vi "Sprache bei den Elementen aendern.vi"(7 "Index":i32, 8 "Fehler (Eingang, kein Fehler)":errorcluster, 9 "Sprachauswahl":u16, 10 "Index verwenden":bool, 11 "VI Referenzen":refnum<vi>[](array[refnum])) -> (0 "Fehler (Ausgang)":errorcluster, 6 "KlassenID":u32[][](array[numeric]))   [LabVIEW 2020, in "Sprachverwaltung.lvlib"]
uses:
  Sprachverwaltung.lvlib
  FGV Aktion Tabelle zerlegen.ctl
panel:
  # "3 Generic \n4 Decoration \n5 Text \n6 Control \n7 ColorBox \n8 Boolean \n9 RefNum \n10 Variant \n11 Path \n12 ListBox \n13 Table \n14 Array \n15 Picture \n16 ActiveXContainer \n17 Numeric \n18 Digital \n19 NamedNumeric \n20 ColorRamp \n21 Slide \n22 GraphOrChart \n23 WaveformChart \n24 WaveformGraph \n25 IntensityChart \n26 IntensityGraph \n27 String \n28 IOName \n29 ComboBox \n30 Cluster \n31 Panel \n32 Knob \n33 NumWithScale \n34 Ring \n35 Enum \n36 GObject \n37 Plot \n38 Cursor \n39 NumericText \n40 Scale \n41 ColorScale \n42 GraphScale \n43 ColorGraphScale \n44 TypedRefNum \n45 OldKnobScale \n46 MCListbox \n47 MeasureData \n48 BVTag \n49 DAQName \n50 VISAName \n51 IVIName \n52 SlideScale \n54 Page \n55 TabControl \n56 ConPane"
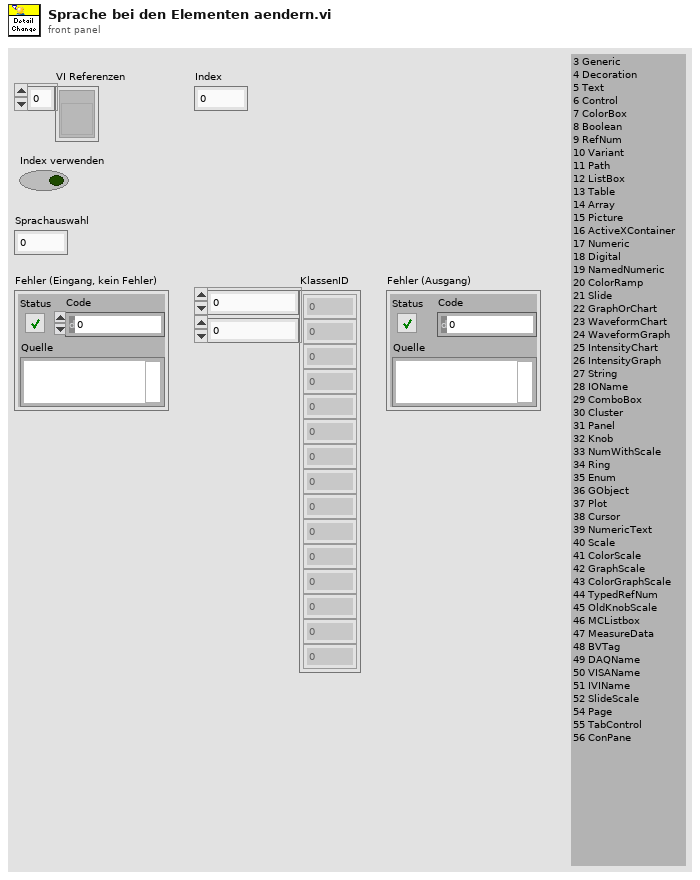
[diagram p1: front panel]
types:
  T1 = typedef "Sprachverwaltung.lvlib/FGV Aktion Tabelle zerlegen.ctl" = enum16{"laden", "vereinzeln", "speichern"}
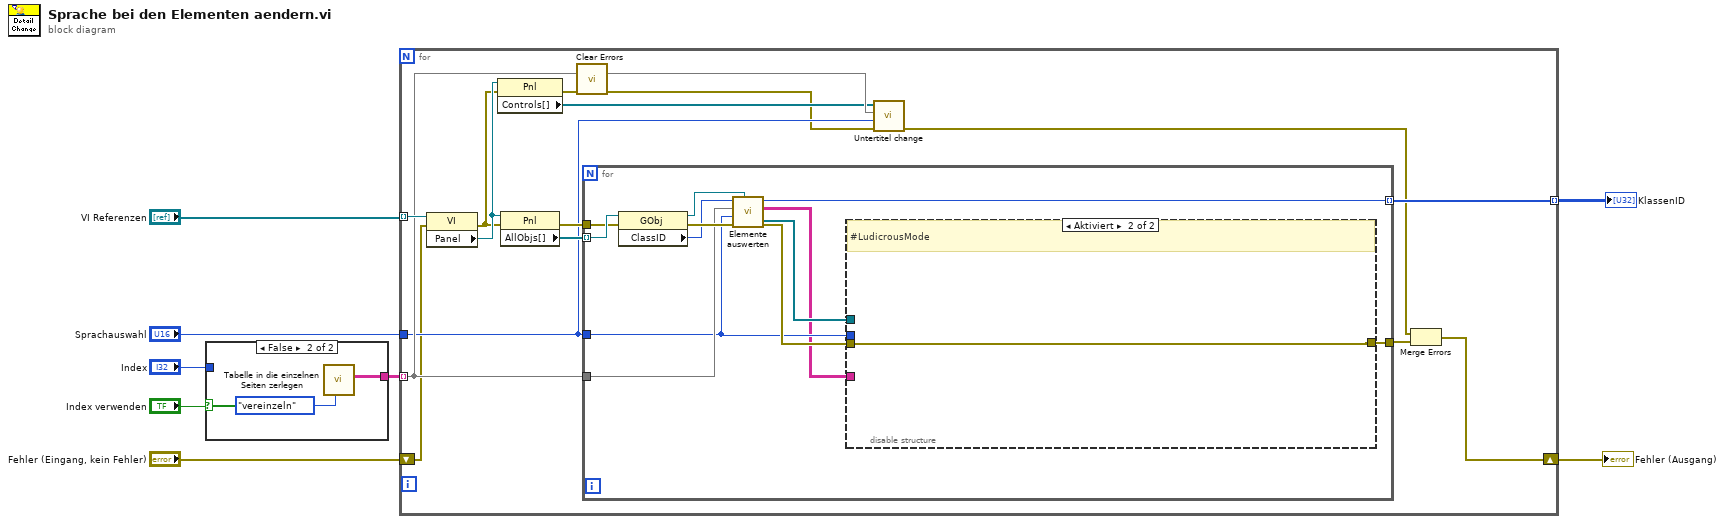
[diagram p0: block diagram]
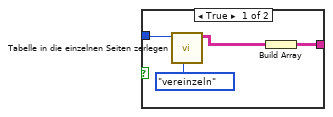
[diagram p2: hidden frame]
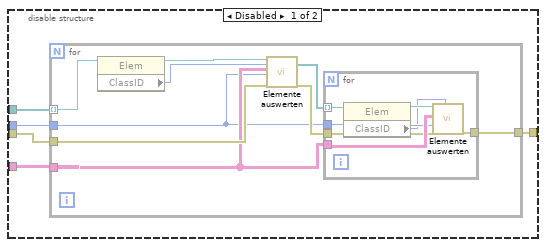
[diagram p3: hidden frame]
diagram:
  n1 = case shown="False" "Index verwenden" {
    tunnel: [w10 w13] -> w6
    tunnel: "Index" -> [w11 _]
    frame True {
      n2 = call "Tabelle in die einzelnen Seiten zerlegen.vi"("Aktion"=FGV_Aktion_Tabelle_zerlegen."vereinzeln", "Index (Seite)"=w11) -> ("Sprachliste"=w9:string[][])  [unwired: 7 in, 2 out]
      n3 = Build Array(w9) -> (w10:string[][][])
    }
    frame False {
      n4 = call "Tabelle in die einzelnen Seiten zerlegen.vi"("Aktion"=FGV_Aktion_Tabelle_zerlegen."vereinzeln") -> ("all rows"=w13:string[][][])  [unwired: 8 in, 2 out]
    }
  }
  n5 = for {
    tunnel: "VI Referenzen" -> [w27] mode=indexing
    tunnel: w6 -> [w25] mode=indexing
    tunnel: "Sprachauswahl" -> [w22]
    tunnel: [w21] -> w3 mode=indexing
    shift-right: [w17] -> w1
    shift-left: "Fehler (Eingang, kein Fehler)" -> [w20]
    n6 = property class="VI"(reference=w27, error in=w20) -> (error out=w24:errorcluster, "Panel"=w26:refnum<vi>)  [unwired: 1 out]
    n7 = property class="Pnl"(reference=w26, error in=w24) -> (error out=w16:errorcluster, "Controls[]"=w23:refnum<vi>[])  [unwired: 1 out]
    n8 = property class="Pnl"(reference=w26, error in=w24) -> (error out=w28:errorcluster, "AllObjs[]"=w29:refnum<vi>[])  [unwired: 1 out]
    n9 = call <vilib>:"Clear Errors.vi"("error in (no error)"=w16) -> ("error out"=w15:errorcluster)  [unwired: 5 in, 1 out]
    n10 = for {
      tunnel: w29 -> [w41] mode=indexing
      tunnel: w25 -> [w36]
      tunnel: w22 -> [w34]
      tunnel: [w32] -> w21 mode=indexing
      tunnel: w28 -> [w39]
      tunnel: [w35] -> w19
      n11 = property class="GObj"(reference=w41, error in=w39) -> (reference out=w31:refnum<vi>, error out=w40:errorcluster, "ClassID"=w33:u32)
      n12 = call "Elemente auswerten.vi"("GObject (Eingang)"=w31, "Fehler (Eingang, kein Fehler)"=w40, "Sprachauswahl"=w34, "all rows"=w36, "ClassID"=w33) -> ("error out"=w37:errorcluster, "all rows out"=w30:string[][], "ClassID out"=w32:u32, "Cluster Elemente[]"=w38:refnum<vi>[])  [unwired: 1 in, 2 out]
      n13 = disable-structure shown="Aktiviert" {
        disable-tunnel: w38 -> [w46 _]
        disable-tunnel: w37 -> [w45 w63]
        disable-tunnel: w30 -> [w44 _]
        disable-tunnel: w34 -> [w43 _]
        disable-tunnel: [w42 w63] -> w35
        frame Disabled {
          n14 = for {
            tunnel: w46 -> [w54] mode=indexing
            tunnel: w44 -> [w51]
            tunnel: w43 -> [w49]
            tunnel: w45 -> [w55]
            tunnel: [w47] -> w42
            n15 = property class="Elem"(reference=w54) -> (reference out=w53:refnum<vi>, "ClassID"=w52:u32)  [unwired: 1 in, 1 out]
            n16 = call "Elemente auswerten.vi"("GObject (Eingang)"=w53, "all rows"=w51, "Sprachauswahl"=w49, "Fehler (Eingang, kein Fehler)"=w55, "ClassID"=w52) -> ("Cluster Elemente[]"=w48:refnum<vi>[], "error out"=w50:errorcluster)  [unwired: 12 in, 1 out]
            n17 = for {
              tunnel: w51 -> [w62]
              tunnel: w50 -> [w61]
              tunnel: w49 -> [w60]
              tunnel: w48 -> [w59] mode=indexing
              tunnel: [w56] -> w47
              n18 = property class="Elem"(reference=w59) -> (reference out=w58:refnum<vi>, "ClassID"=w57:u32)  [unwired: 1 in, 1 out]
              n19 = call "Elemente auswerten.vi"("GObject (Eingang)"=w58, "all rows"=w62, "Sprachauswahl"=w60, "Fehler (Eingang, kein Fehler)"=w61, "ClassID"=w57) -> ("error out"=w56:errorcluster)  [unwired: 12 in, 2 out]
            }
          }
        }
        frame Enabled {
          # "#LudicrousMode"
        }
      }
    }
    n20 = call "Untertitel change.vi"("Fehler (Eingang, kein Fehler)"=w15, "Sprachauswahl"=w22, "Sprachdatei"=w25, "Controls[]"=w23) -> ("Fehler (Ausgang, kein Fehler)"=w18:errorcluster)  [unwired: 5 in, 2 out]
    n21 = Merge Errors(w18, w19) -> (w17:errorcluster)
  }
  "Fehler (Ausgang)" <- w1
  "KlassenID" <- w3
